vi "init.vi"(8 "error in":errorcluster, 10 "TBM module configuration in":refnum<class "TBM module configuration.lvclass">, 11 "TDMS datalogger runtime in":refnum<class "TDMS datalogger runtime.lvclass">) -> (0 "error out":errorcluster, 1 "data allocations":T1, 2 "execution settings":T4, 3 "TDMS datalogger runtime out":refnum<class "TDMS datalogger runtime.lvclass">)   [LabVIEW 2013, in "TDMS datalogger runtime.lvclass"]
doc: "Provides an interface for initializing a module at runtime. While this interface performs no operations, a child should provide an override which may open any necessary references or sessions, allocate necessary memory, and perform any final configuration validataion before providing the full configuration <b>execution data</b> to the calling process."
uses:
  TDMS datalogger runtime.lvclass
  <vilib>/NI/Tag Bus Module Framework/channel/TBM channel.lvclass
  <vilib>/NI/Tag Bus Module Framework/runtime/TBM module execution interface.lvclass
  configuration/TDMS datalogger configuration.lvclass
  <vilib>/NI/Tag Bus Module Framework/runtime/execution settings.ctl
  <vilib>/NI/Tag Bus/dictionary/data dictionary.lvclass
  control enum.ctl
  <vilib>/NI/Tag Bus/table/data table.ctl
  <vilib>/NI/Tag Bus/table/data table.lvlib
  sample queue.ctl
  <vilib>/NI/Tag Bus Module Framework/module configuration/TBM module configuration.lvclass
  <vilib>/NI/Tag Bus Module Framework/channel/data tables.ctl
  <vilib>/NI/Tag Bus/dictionary table pair.ctl
  <vilib>/NI/Tag Bus/tag bus.lvlib
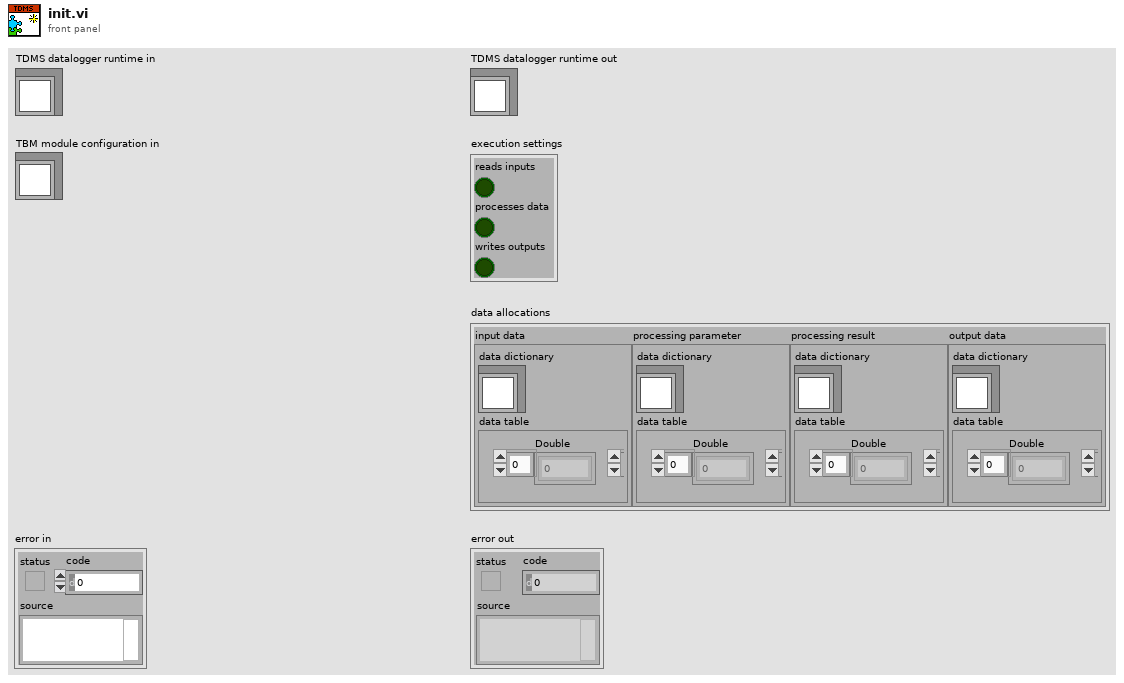
[diagram p1: front panel]
types:
  T1 = typedef "TBM channel.lvclass/data tables.ctl" = cluster{"input data":T2, "processing parameter":T2, "processing result":T2, "output data":T2}
  T2 = typedef "tag bus.lvlib/dictionary table pair.ctl" = cluster{"data dictionary":refnum<class "data dictionary.lvclass">, "data table":T3}
  T3 = typedef "tag bus.lvlib/data table.lvlib/data table.ctl" = cluster{"Double":dbl[], "Single":sgl[], "I64":i64[], "I32":i32[], "I16":i16[], "I8":i8[], "U64":u64[], "U32":u32[], "U16":u16[], "U8":u8[], "Boolean":bool[], "String":string[], "Array of Double":cluster{"DBL Array":dbl[]}[], "Array of Single":cluster{"SGL Array":sgl[]}[], "Array of I64":cluster{"I64 Array":i64[]}[], "Array of I32":cluster{"I32 Array":i32[]}[], "Array of I16":cluster{"I16 Array":i16[]}[], "Array of I8":cluster{"I8 Array":i8[]}[], "Array of U64":cluster{"U64 Array":u64[]}[], "Array of U32":cluster{"U32 Array":u32[]}[], "Array of U16":cluster{"U16 Array":u16[]}[], "Array of U8":cluster{"U8 Array":u8[]}[], "Array of Boolean":cluster{"Boolean Array":bool[]}[], "Array of String":cluster{"String Array":string[]}[]}
  T4 = typedef "TBM module execution interface.lvclass/execution settings.ctl" = cluster{"reads inputs":bool, "processes data":bool, "writes outputs":bool}
  T5 = typedef "TDMS datalogger runtime.lvclass/sample queue.ctl" = cluster{"data to processor":refnum<queue>, "time to processor":refnum<queue>}
  T6 = typedef "TDMS datalogger runtime.lvclass/control enum.ctl" = enum16{"exit"}
  T7 = typedef "tag bus.lvlib/tag descriptor.lvclass/Data Type.ctl" = enum16{"Double", "Single", "I64", "I32", "I16", "I8", "U64", "U32", "U16", "U8", "Boolean", "String", "Array of Double", "Array of Single", "Array of I64", "Array of I32", "Array of I16", "Array of I8", "Array of U64", "Array of U32", "Array of U16", "Array of U8", "Array of Boolean", "Array of String"}
  T8 = typedef "tag bus.lvlib/data dictionary.lvclass/full data dictionary.ctl" = cluster{"Double":string[], "Single":string[], "I64":string[], "I32":string[], "I16":string[], "I8":string[], "U64":string[], "U32":string[], "U16":string[], "U8":string[], "Boolean":string[], "String":string[], "Array of Double":string[], "Array of Single":string[], "Array of I64":string[], "Array of I32":string[], "Array of I16":string[], "Array of I8":string[], "Array of U64":string[], "Array of U32":string[], "Array of U16":string[], "Array of U8":string[], "Array of Boolean":string[], "Array of String":string[]}
  T9 = typedef "tag bus.lvlib/data table.lvlib/allocation specification.ctl" = cluster{"data type":T7, "size":i32}
  T10 = typedef "TDMS datalogger runtime.lvclass/data cache.ctl" = cluster{"timestamps":timestamp[], "Double":dbl[][], "Single":sgl[][], "I64":i64[][], "I32":i32[][], "I16":i16[][], "I8":i8[][], "U64":u64[][], "U32":u32[][], "U16":u16[][], "U8":u8[][], "Boolean":bool[][]}
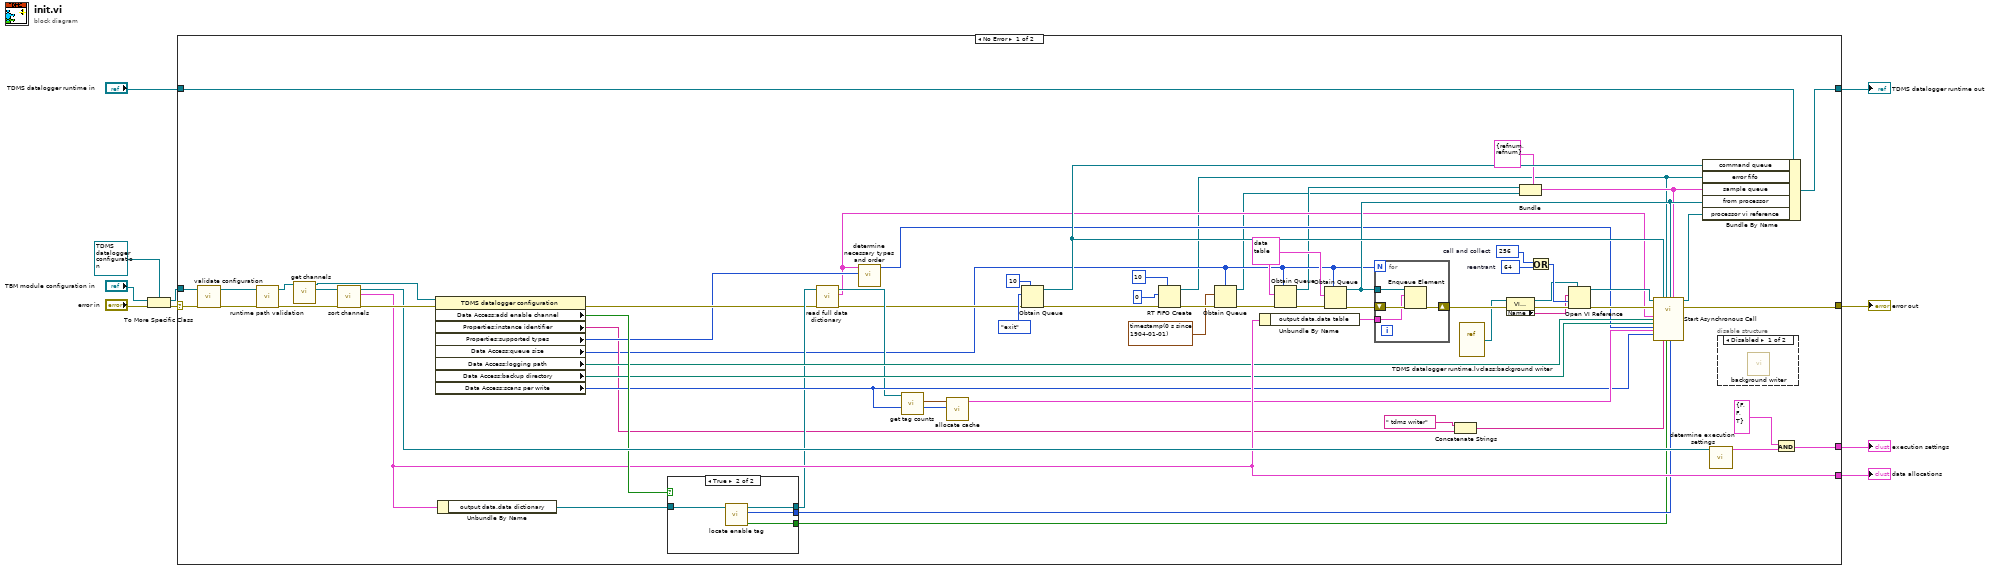
[diagram p0: block diagram]
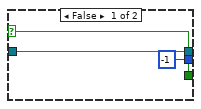
[diagram p2: hidden frame]
diagram:
  n1 = To More Specific Class(target class=refnum<class "TDMS datalogger configuration.lvclass"> refnum ("Synchronous module configuration"), reference="TBM module configuration in", error in="error in") -> (specific class reference=w9:refnum<class "TDMS datalogger configuration.lvclass">, error out=w10:errorcluster)
  n2 = case shown="No Error" w10 {
    selector: w10 -> [w73 w89]
    tunnel: w9 -> [w72 _]
    tunnel: "TDMS datalogger runtime in" -> [w71 w90]
    tunnel: [w70 w90] -> w4
    tunnel: [w55 w89] -> w3
    tunnel: [w48 _] -> w1
    tunnel: [w66 _] -> w2
    frame No Error {
      w46 = T3 {"Double"=[], "Single"=[], "I64"=[], "I32"=[], "I16"=[], "I8"=[], "U64"=[], "U32"=[], "U16"=[], "U8"=[], "Boolean"=[], "String"=[], "Array of Double"=[], "Array of Single"=[], "Array of I64"=[], "Array of I32"=[], "Array of I16"=[], "Array of I8"=[], "Array of U64"=[], "Array of U32"=[], "Array of U16"=[], "Array of U8"=[], "Array of Boolean"=[], "Array of String"=[]} ("Data Interface out")
      w61 = 64  # reentrant
      w60 = 256  # call and collect
      n3 = call-dynamic "validate configuration.vi"("error in"=w73, "TDMS datalogger configuration in"=w72) -> ("error out"=w74:errorcluster, "TDMS datalogger configuration out"=w18:refnum<class "TDMS datalogger configuration.lvclass">)  [unwired: 8 in]
      n4 = call "runtime path validation.vi"("error in"=w74, "TDMS datalogger configuration in"=w18) -> ("error out"=w19:errorcluster, "TDMS datalogger configuration out"=w17:refnum<class "TDMS datalogger configuration.lvclass">)  [unwired: 8 in]
      n5 = call-dynamic "get channels.vi"("module configuration in"=w17) -> ("channels"=w15:refnum<class "TBM channel.lvclass">[], "module configuration out"=w16:refnum<class "TDMS datalogger configuration.lvclass">)  [unwired: 9 in]
      n6 = call <vilib>:"sort channels.vi"("error in"=w19, "channels in"=w15) -> ("error out"=w77:errorcluster, "data allocations"=w48:T1, "channels out"=w75:refnum<class "TBM channel.lvclass">[])  [unwired: 7 in]
      n7 = property class="TDMS datalogger configuration"(reference=w16, error in=w77) -> (error out=w36:errorcluster, "Data Access:add enable channel"=w53:bool, "Properties:instance identifier"=w31:string, "Properties:supported types"=w35:T7[], "Data Access:queue size"=w24:i32, "Data Access:logging path"=w43:path, "Data Access:backup directory"=w42:path, "Data Access:scans per write"=w41:i32)  [unwired: 1 out]
      n8 = Unbundle By Name(w48) -> ("output data.data dictionary"=w54:refnum<class "data dictionary.lvclass">)
      n9 = case shown="True" w53 {
        selector: w53 -> [w80 _]
        tunnel: w54 -> [w79 w84]
        tunnel: [w79 w83] -> w38
        tunnel: [w80 w81] -> w27
        tunnel: [-1 ("index") w82] -> w28
        frame False {
        }
        frame True {
          n10 = call "locate enable tag.vi"("data dictionary in"=w84) -> ("found?"=w81:bool, "index"=w82:i32, "data dictionary out"=w83:refnum<class "data dictionary.lvclass">)  [unwired: 8 in]
        }
      }
      n11 = call <vilib>:"read full data dictionary.vi"("error in"=w36, "data dictionary in"=w38) -> ("error out"=w34:errorcluster, "dictionary"=w33:T8, "data dictionary out"=w37:refnum<class "data dictionary.lvclass">)  [unwired: 7 in]
      n12 = call "determine necessary types and order.vi"("supported types"=w35, "dictionary"=w33) -> ("output type order"=w32:T7[])  [unwired: 9 in]
      n13 = call <vilib>:"get tag counts.vi"("data dictionary in"=w37) -> ("counts"=w64:T9[])  [unwired: 9 in, 1 out]
      n14 = call "allocate cache.vi"("scans per write"=w41, "counts"=w64) -> ("cache allocation"=w44:T10)  [unwired: 9 in]
      n15 = Obtain Queue(max queue size (-1, unlimited)=10, element data type=control_enum."exit" ("control enum"), error in (no error)=w34) -> (queue out=w49:refnum<queue>, error out=w52:errorcluster)  [unwired: 2 in, 1 out]
      n16 = RT FIFO Create(1:0, 3:w52, 4:u32 10 ("size (10)")) -> (8:w12:refnum<k33>, 11:w67:errorcluster)  [unwired: 5 in, 1 out]
      n17 = Obtain Queue(max queue size (-1, unlimited)=w24, element data type=timestamp(0 s since 1904-01-01), error in (no error)=w67) -> (queue out=w20:refnum<queue>, error out=w26:errorcluster)  [unwired: 2 in, 1 out]
      n18 = Unbundle By Name(w48) -> ("output data.data table"=w47:T3)
      n19 = Obtain Queue(max queue size (-1, unlimited)=w24, element data type=w46, error in (no error)=w26) -> (queue out=w21:refnum<queue>, error out=w68:errorcluster)  [unwired: 2 in, 1 out]
      n20 = Obtain Queue(max queue size (-1, unlimited)=w24, element data type=w46, error in (no error)=w68) -> (queue out=w39:refnum<queue>, error out=w69:errorcluster)  [unwired: 2 in, 1 out]
      n21 = for {
        N: w24 -> [_]
        shift-right: [w87] -> w57
        shift-left: w69 -> [w88]
        tunnel: w39 -> [w86]
        tunnel: w47 -> [w85]
        n22 = Enqueue Element(queue=w86, element=w85, error in (no error)=w88) -> (error out=w87:errorcluster)  [unwired: 1 in, 2 out]
      }
      n23 = Concatenate Strings(" tdms writer" ("string"), w31) -> (w30:string)
      n24 = vi-ref "TDMS datalogger runtime.lvclass:background writer.vi"() -> (w56:refnum<vi>)
      n25 = property class="VI (strict)"(reference=w56, error in=w57) -> (reference out=w14:refnum<vi>, error out=w59:errorcluster, "Name"=w58:string)
      n26 = Bundle(cluster=T5 {"data to processor"=refnum, "time to processor"=refnum} ("sample queue"), "data to processor"=w21, "time to processor"=w20) -> (w22:T5)
      n27 = Or(x=w60, y=w61) -> (x .or. y?=w62:i32)
      n28 = Open VI Reference(type specifier VI Refnum (for type only)=w14, vi path=w58, options=w62, error in (no error)=w59) -> (vi reference=w45:refnum<vi>, error out=w63:errorcluster)  [unwired: 2 in]
      n29 = call-by-ref "Start Asynchronous Call"(reference=w45, error in=w63, "dictionary"=w33, "logging path"=w43, "backup directory"=w42, "output type order"=w32, "cache allocation"=w44, "scans per write"=w41, "command queue"=w49, "group name"=w30, "error fifo"=w12, "has enable channel"=w27, "from background"=w39, "enable channel (bool)"=w28, "sample queue"=w22) -> (reference out=w40:refnum<vi>, error out=w55:errorcluster)  [unwired: 6 in, 1 out]
      n30 = Bundle By Name(cluster=w71, "command queue"=w49, "error fifo"=w12, "sample queue"=w22, "from processor"=w39, "processor vi reference"=w40) -> (w70:refnum<class "TDMS datalogger runtime.lvclass">)
      n31 = call <vilib>:"determine execution settings.vi"("channels"=w75) -> ("execution settings"=w76:T4)  [unwired: 10 in]
      n32 = disable-structure shown="Disabled" {
        frame Disabled {
          n33 = call "background writer.vi"() -> ()  [unwired: 19 in, 1 out]
        }
        frame Enabled {
        }
      }
      n34 = And(x=T4 {"reads inputs"=FALSE, "processes data"=FALSE, "writes outputs"=TRUE}, y=w76) -> (x .and. y?=w66:T4)
    }
    frame Error {
    }
  }
  "error out" <- w3
  "TDMS datalogger runtime out" <- w4
  "execution settings" <- w2
  "data allocations" <- w1
